vi "OvenControlPanel.vi"() -> ()   [LabVIEW 2023]
uses:
  <vilib>/numeric/Random Number (Range) I64.vi
  <vilib>/numeric/sub_Random U32.vi
panel:
  in  "file path (use dialog)":path
  out "Elapsed Time (s)":i64
  out "Waveform Chart":waveform(i64)(graph)={"t0"=timestamp(3782760733.4076047 s since 1904-01-01), "dt"=1.0, "Y"=[24]}
  out "Current Temperature":i64
  in  "Set Warnings Limit":T1
  in  "Time Target (s)":dbl=10.0
  out "Warning":string
  out "Boolean":bool
  in  "stop":bool
  out "Current Board":string
  in  "Select Board For Test":string(combo)
  # "Please select logfile path before start (create it)"
  # "Please select Min and Max value for Temp"
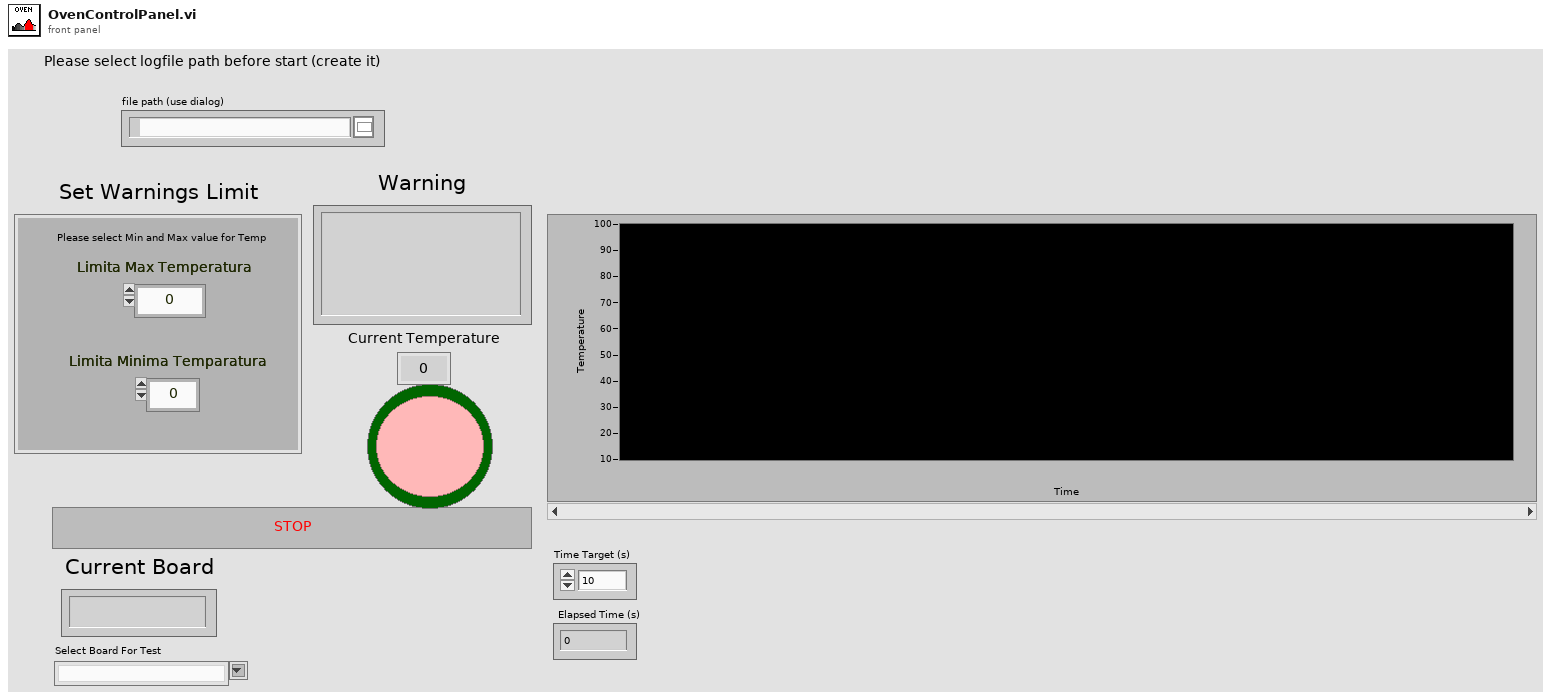
[diagram p1: front panel]
types:
  T1 = cluster{"Limita Max Temperatura":dbl, "Limita Minima Temparatura":dbl}
  T2 = enum16{"open", "replace", "create", "open or create", "replace or create", "replace or create with confirmation"}
  T3 = typedef "imagedata.ctl" = cluster{"image type":i32, "image depth":i32, "image":u8[], "mask":u8[], "colors":u32[], "Rectangle":cluster{"left":i16, "top":i16, "right":i16, "bottom":i16}}
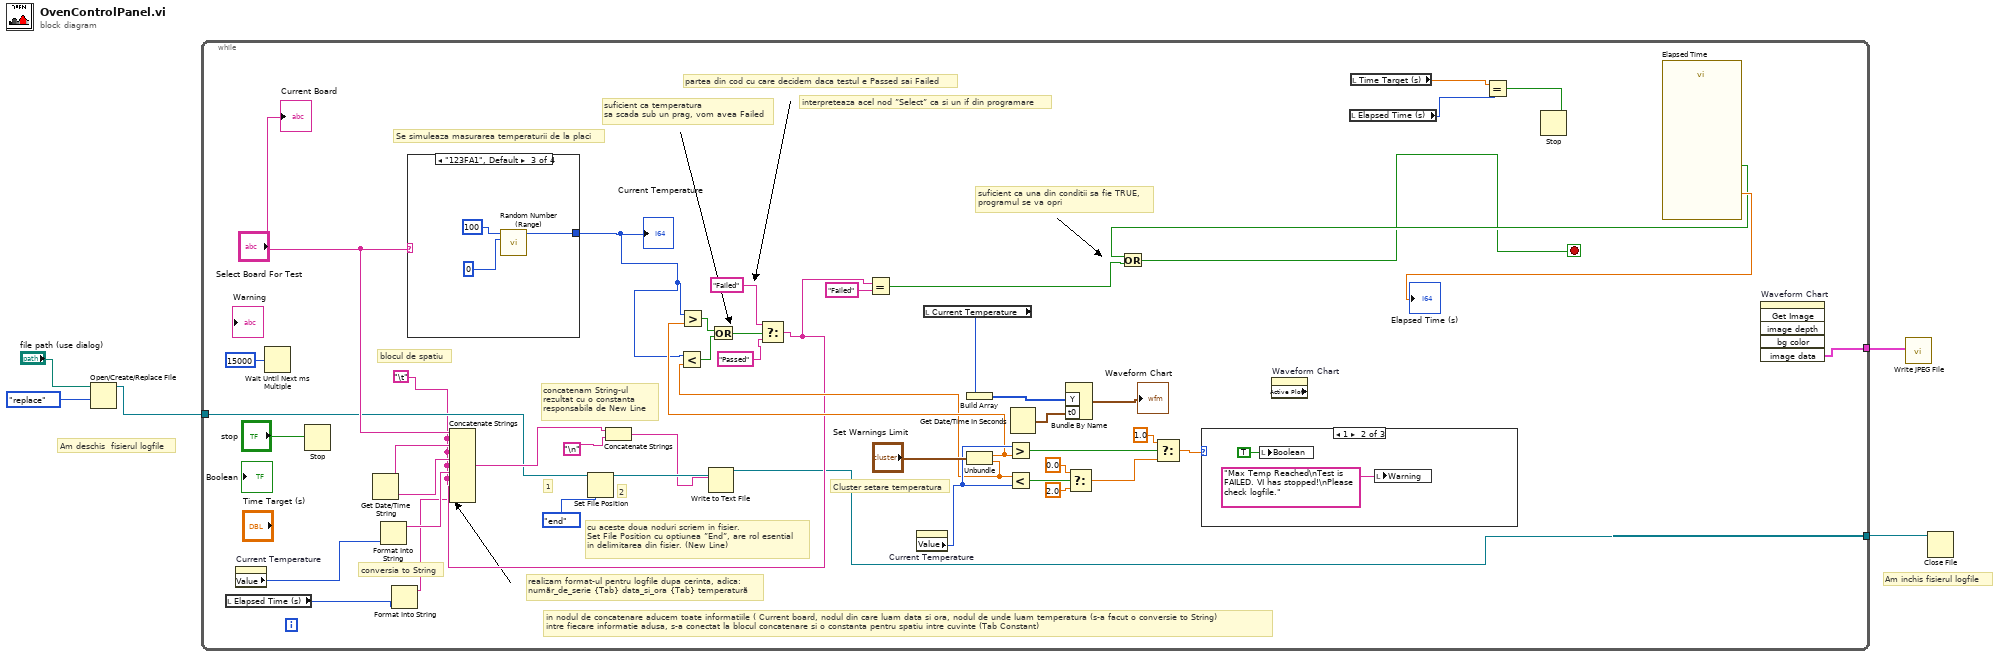
[diagram p0: block diagram]
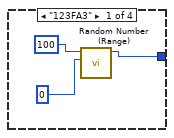
[diagram p2: hidden frame]
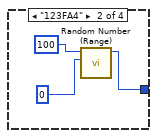
[diagram p3: hidden frame]
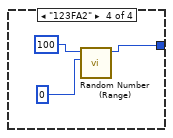
[diagram p4: hidden frame]
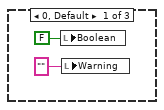
[diagram p5: hidden frame]
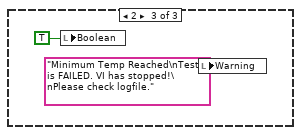
[diagram p6: hidden frame]
diagram:
  # "Am inchis fisierul logfile"
  # "Am deschis  fisierul logfile"
  n1 = Open/Create/Replace File(file path (use dialog)="file path (use dialog)", operation (0:open)=T2."replace") -> (refnum out=w3:refnum<file>)  [unwired: 4 in, 2 out]
  n2 = while {
    tunnel: [w8] -> w5
    tunnel: w3 -> [w14]
    tunnel: [w13] -> w1
    stop <- w15 stop-if-true
    w11 = "\t" ("Tab Constant")
    # "Cluster setare temperatura"
    # "suficient ca temperatura\nsa scada sub un prag, vom avea Failed"
    # "interpreteaza acel nod ”Select” ca si un if din programare"
    # "partea din cod cu care decidem daca testul e Passed sai Failed"
    # "suficient ca una din conditii sa fie TRUE,\nprogramul se va opri"
    # "concatenam String-ul rezultat cu o constanta\nresponsabila de New Line"
    # "3"
    # "2"
    # "1"
    # "cu aceste doua noduri scriem in fisier.\nSet File Position cu optiunea ”End”, are rol esential\nin delimitarea din fisier. (New Line)"
    # "blocul de spatiu"
    # "conversia to String"
    # "in nodul de concatenare aducem toate informatiile ( Current board, nodul din care luam data si ora, nodul de unde luam temperatura (s-a facut o conversie to String)\nintre fiecare informatie adusa, s-a conectat la blocul concatenare si o constanta pentru spatiu intre cuvinte (Tab Constant)"
    # "realizam format-ul pentru logfile dupa cerinta, adica: \nnumãr_de_serie {Tab} data_si_ora {Tab} temperaturã"
    # "Se simuleaza masurarea temperaturii de la placi"
    n3 = local read "Elapsed Time (s)"() -> (w10:i64)
    n4 = property on="Current Temperature" class="DigNum (strict)"() -> ("Value"=w28:i64)  [unwired: 2 in, 2 out]
    n5 = Wait Until Next ms Multiple(millisecond multiple=u32 15000) -> ()  [unwired: 1 out]
    n6 = Stop(stop? (T)="stop") -> ()
    n7 = Get Date/Time String() -> (date string=w39:string, time string=w38:string)  [unwired: 3 in]
    n8 = Format Into String "Format Into String"(w28) -> (resulting string=w27:string)  [unwired: 3 in, 1 out]
    n9 = Format Into String "Format Into String"(w10) -> (resulting string=w9:string)  [unwired: 3 in, 1 out]
    n10 = case shown="\"123FA1\", Default" "Select Board For Test" {
      tunnel: [w54 w57 w60 w63] -> w22
      frame "123FA3" {
        n11 = call-poly <vilib>:"Random Number (Range).vi"("lower bound (-100)"=u64 0 ("lower bound (0)"), "upper bound (100)"=u64 100) -> ("number"=w54:i64)  [unwired: 9 in]
      }
      frame "123FA4" {
        n12 = call-poly <vilib>:"Random Number (Range).vi"("lower bound (-100)"=u64 0 ("lower bound (0)"), "upper bound (100)"=u64 100) -> ("number"=w57:i64)  [unwired: 9 in]
      }
      frame "123FA1", Default {
        n13 = call-poly <vilib>:"Random Number (Range).vi"("lower bound (-100)"=u64 0 ("lower bound (0)"), "upper bound (100)"=u64 100) -> ("number"=w60:i64)  [unwired: 9 in]
      }
      frame "123FA2" {
        n14 = call-poly <vilib>:"Random Number (Range).vi"("lower bound (-100)"=u64 0 ("lower bound (0)"), "upper bound (100)"=u64 100) -> ("number"=w63:i64)  [unwired: 9 in]
      }
    }
    "Current Temperature" <- w22
    n15 = Set File Position(refnum=w14, from (0:start)=enum16{"start", "end", "current"}."end") -> (refnum out=w37:refnum<file>)  [unwired: 2 in, 1 out]
    n16 = property on="Current Temperature" class="DigNum (strict)"() -> ("Value"=w33:i64)  [unwired: 2 in, 2 out]
    n17 = local read "Current Temperature"() -> (w6:i64)
    n18 = Build Array(w6) -> (w48:i64[])
    n19 = Unbundle("Set Warnings Limit") -> ("Limita Max Temperatura"=w23:dbl, "Limita Minima Temparatura"=w21:dbl)
    n20 = Less?(x=w22, y=w21) -> (x < y?=w31:bool)
    n21 = Greater?(x=w22, y=w23) -> (0:w32:bool)
    n22 = Or(x=w32, y=w31) -> (x .or. y?=w30:bool)
    n23 = Select(t="Failed" ("String"), s=w30, f="Passed" ("String")) -> (s? t:f=w17:string)
    n24 = Concatenate Strings "Concatenate Strings"("Select Board For Test", w11, w39, w11, w38, w11, w27, w11, w17, w11, w9) -> (w26:string)
    n25 = Concatenate Strings(w26, "\n" ("Line Feed Constant")) -> (w24:string)
    n26 = Write to Text File(file (use dialog)=w37, text=w24) -> (refnum out=w8:refnum<file>)  [unwired: 2 in, 2 out]
    n27 = Equal?(x=w17, y="Failed") -> (x = y?=w16:bool)
    n28 = Greater?(x=w33, y=w23) -> (0:w34:bool)
    n29 = Less?(x=w21, y=w33) -> (x < y?=w35:bool)
    n30 = Get Date/Time In Seconds() -> (seconds since 1Jan1904=w50:timestamp)
    n31 = Bundle By Name ("Build Waveform")("Y"=w48, "t0"=w50) -> (→"Waveform Chart":waveform(i64))  [unwired: 1 in]
    n32 = Select(t=0.0, s=w35, f=2.0) -> (s? t:f=w46:dbl)
    n33 = Select(t=1.0, s=w34, f=w46) -> (s? t:f=w49:dbl)
    n34 = case shown="1" w49 {
      frame 0, Default {
        n35 = local write "Boolean"(FALSE ("Boolean")) -> ()
        n36 = local write "Warning"("") -> ()
      }
      frame 1 {
        n37 = local write "Boolean"(TRUE ("Boolean")) -> ()
        n38 = local write "Warning"("Max Temp Reached\nTest is FAILED. VI has stopped!\nPlease check logfile.") -> ()
      }
      frame 2 {
        n39 = local write "Boolean"(TRUE ("Boolean")) -> ()
        n40 = local write "Warning"("Minimum Temp Reached\nTest is FAILED. VI has stopped!\nPlease check logfile.") -> ()
      }
    }
    n41 = property on="Waveform Chart" class="WFChart (strict)" props=["Active Plot"]() -> ()  [unwired: 2 in, 3 out]
    n42 = local read "Elapsed Time (s)"() -> (w51:i64)
    n43 = local read "Time Target (s)"() -> (w52:dbl)
    n44 = Equal?(x=w52, y=w51) -> (x = y?=w12:bool)
    n45 = Stop(stop? (T)=w12) -> ()
    n46 = call "Elapsed Time"() -> ("Elapsed Time (s)"=→"Elapsed Time (s)":dbl, "Time has Elapsed"=w20:bool)  [unwired: 12 in, 6 out]
    n47 = Or(x=w20, y=w16) -> (x .or. y?=w15:bool)
    n48 = invoke on="Waveform Chart" class="WFChart (strict)" method="Get Image"() -> ("image data"=w13:T3)  [unwired: 6 in, 5 out]
    "Current Board" <- "Select Board For Test"
  }
  n49 = call <vilib>:"Write JPEG File.vi"("image data"=w1) -> ()  [unwired: 9 in, 2 out]
  n50 = Close File(refnum=w5) -> ()  [unwired: 1 in, 2 out]
